vi "LAS-CTS_TargetScanner.vi"() -> ()   [LabVIEW 2024]
doc: "Shows how to move a motor to an absolute position."
uses:
  E:/E-book/LAS/LAS DAQ/LAS LV Scan/Kinesis/Thorlabs.MotionControl.Controls.dll
  Kinesis/Thorlabs.MotionControl.Controls.dll
  <vilib>/Analysis/baseanly.llb/Mean (DBL).vi
  E:/E-book/LAS/LAS DAQ/LAS LV Scan/Kinesis/ThorLabs.MotionControl.KCube.DCServoCLI.dll
  Kinesis/ThorLabs.MotionControl.KCube.DCServoCLI.dll
  <vilib>/httpClient/LabVIEWHTTPClient.lvlib
  <vilib>/Analysis/NI_AALBase.lvlib
panel:
  out "Filename":path
  in  "File #":i32 format="%03d"
  in  "base filename":string
  in  "Filepath":path
  in  "Target ID":string
  out "Last Spot Charge (pC)":dbl
  out "Laser Energy (uJ)":dbl format="%#.3f"
  out "Pulses Remaining":i32
  out "Laser On/Off":bool
  in  "Energy Meter VISA port":refnum<visa-resource-name>="IntegraEnergyMeter"
  in  "Keithley VISA port":refnum<visa-resource-name>="Keithly6514"
  out "Scan Graph":dbl[][](graph)
  in  "KCubeDCServoControl Z axis":refnum<k24>(container)
  in  "KCubeDCServoControl X axis":refnum<k24>(container)
  out "K6514 Error":errorcluster
  out "Time Remaining (min)":dbl format="%#_2f"
  out "sec per spot":dbl
  out "scan started":bool
  out "Scan Progress":u8(slide) scale=0.0..42.0
  out "Scan Time (hr)":dbl format="%#_2f"
  in  "Number of Laser Pulses":i32=100
  in  "X Start Position":dbl=5.0
  in  "Z Start Position":dbl=4.0
  in  "Z Step Size (um)":dbl=500.0
  in  "# of Z Positions":i32=2
  in  "# of X Positions":i32=2
  in  "X Step Size (um)":dbl=500.0
  in  "Start Scan":bool
  out "CurrentPosZ":dbl=6.0
  out "CurrentPosX":dbl=6.0
  in  "SerialNumber Z":string="27261646"
  in  "SerialNumber X":string="27261828"
  # "Connection Setup"
  # "Scan Parameters"
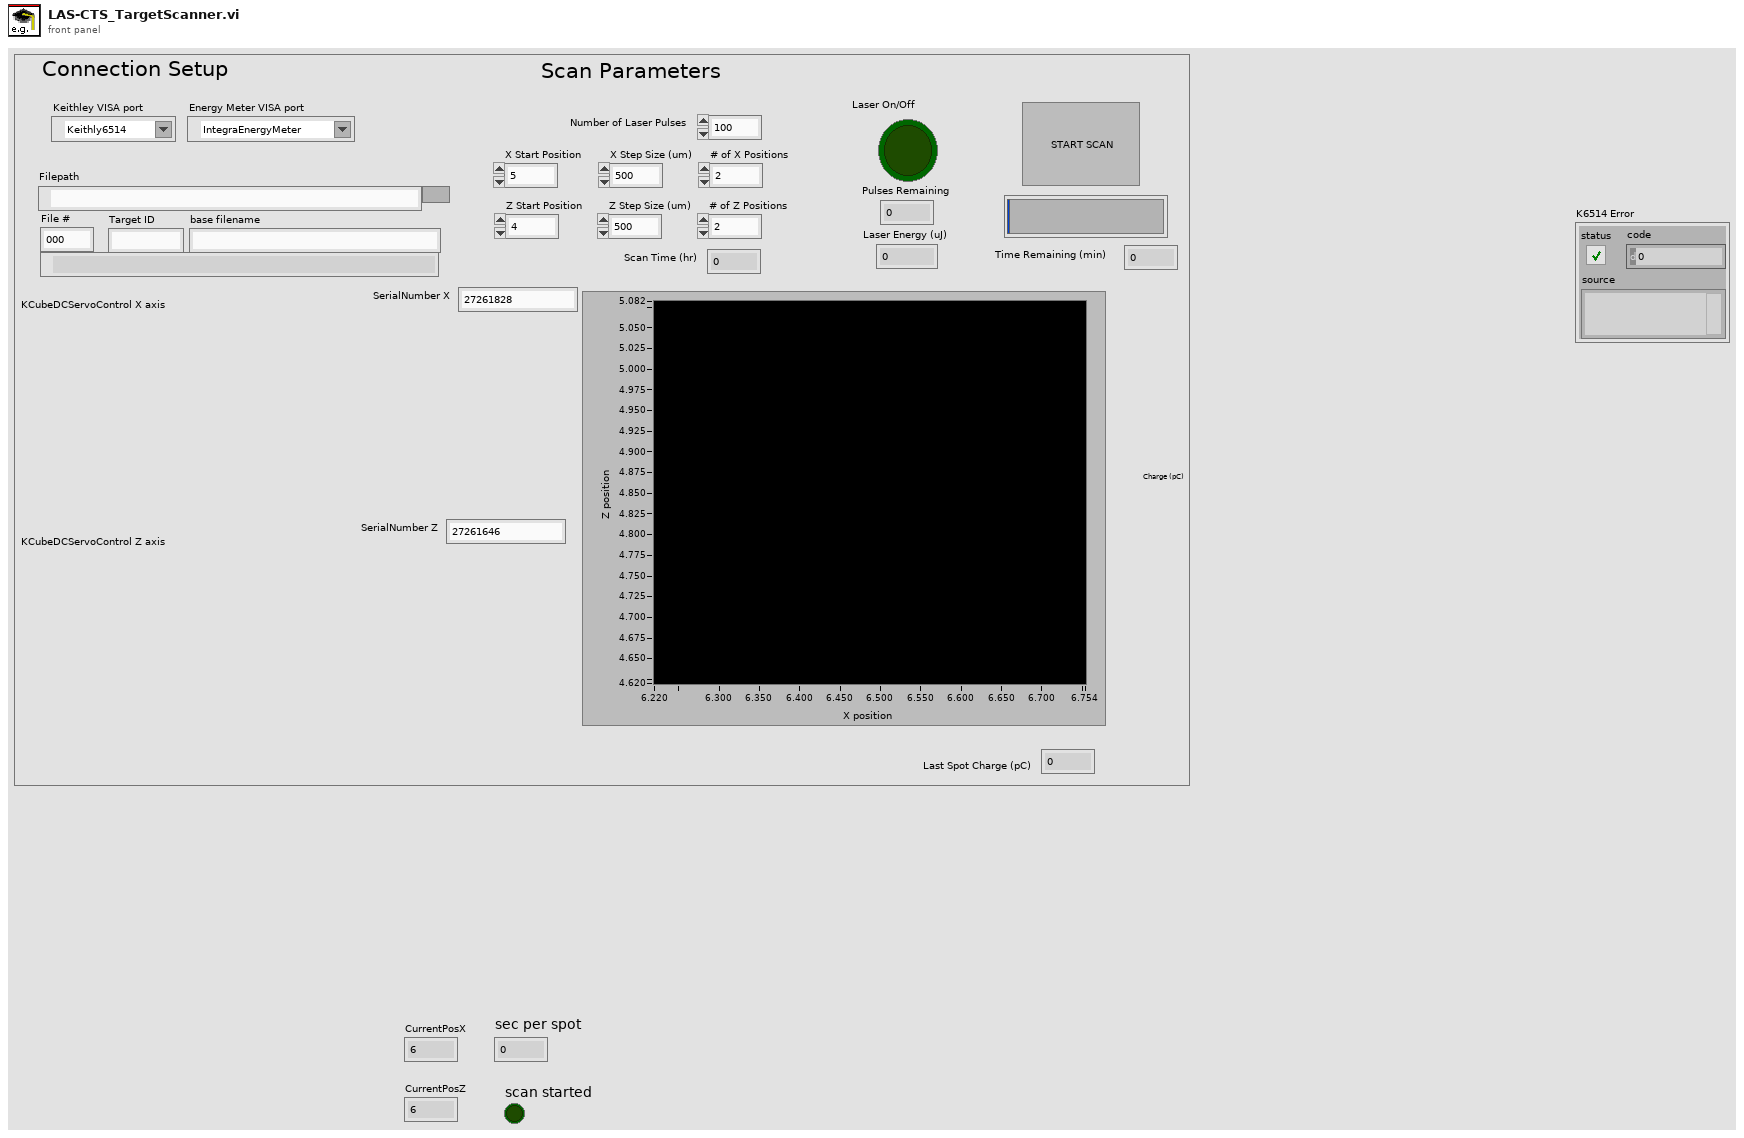
[diagram p1: front panel]
types:
  T1 = enum16{"open", "replace", "create", "open or create", "replace or create", "replace or create with confirmation"}
  T2 = typedef "LabVIEWHTTPClient.lvlib/ClientHandle.ctl" = refnum<k1>
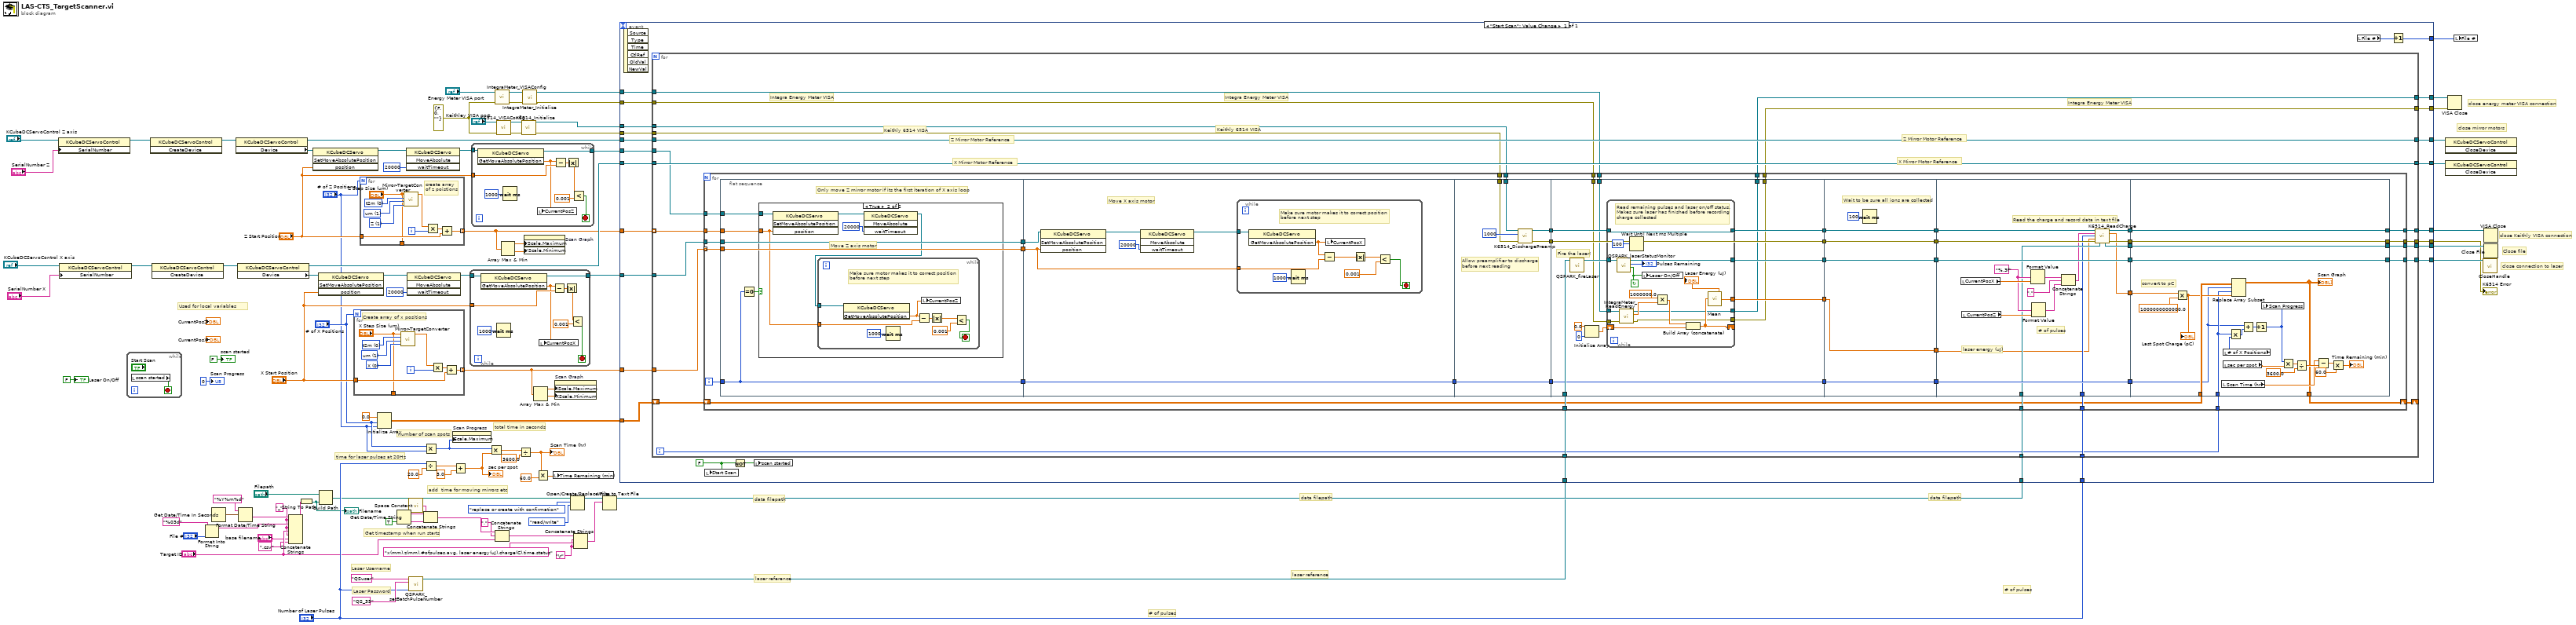
[diagram p0: block diagram]
diagram:
  w7 = "_" ("string")
  w32 = errorcluster {"status"=FALSE, "code"=0, "source"=""} ("error in (no error)")
  w25 = "\r"
  # "Get timestamp when run starts"
  # "close energy meter VISA connection"
  # "total time in seconds"
  # "add  time for moving mirrors etc"
  # "number of scan spots"
  # "time for laser pulses at 20Hz"
  # "data filepath"
  # "data filepath"
  # "close Keithly VISA connection"
  # "close mirror motors"
  # "close connection to laser"
  # "Close file"
  # "Used for local variables"
  # "data filepath"
  # "laser reference"
  # "# of pulses"
  # "# of pulses"
  # "laser reference"
  # "Laser Password"
  # "Laser Username"
  n1 = property class="KCubeDCServoControl"(reference="KCubeDCServoControl Z axis", "SerialNumber"="SerialNumber Z") -> (reference out=w94:refnum<k24>)  [unwired: 1 in, 1 out]
  n2 = property class="KCubeDCServoControl"(reference="KCubeDCServoControl X axis", "SerialNumber"="SerialNumber X") -> (reference out=w97:refnum<k24>)  [unwired: 1 in, 1 out]
  n3 = while {
    stop <- w98 stop-if-true
    n4 = local read "scan started"() -> (w98:bool)
  }
  n5 = invoke class="KCubeDCServoControl" method="CreateDevice"(reference=w94) -> (reference out=w88:refnum<k24>)  [unwired: 2 in, 2 out]
  n6 = invoke class="KCubeDCServoControl" method="CreateDevice"(reference=w97) -> (reference out=w95:refnum<k24>)  [unwired: 2 in, 2 out]
  n7 = Format Into String(format string="%03d", "File #") -> (resulting string=w10:string)  [unwired: 2 in, 1 out]
  n8 = Get Date/Time In Seconds() -> (seconds since 1Jan1904=w15:timestamp)
  n9 = property class="KCubeDCServoControl"(reference=w88) -> (reference out=w85:refnum<k24>, "Device"=w1:refnum<k24>)  [unwired: 1 in, 1 out]
  n10 = property class="KCubeDCServoControl"(reference=w95) -> (reference out=w84:refnum<k24>, "Device"=w76:refnum<k24>)  [unwired: 1 in, 1 out]
  n11 = Format Date/Time String(time format string (%c)="%Y%m%d", seconds (now)=w15) -> (date/time string=w13:string)  [unwired: 1 in]
  n12 = Concatenate Strings(w13, w7, w10, w7, "Target ID", w7, "base filename", ".csv" ("string")) -> (w16:string)
  n13 = String To Path(string=w16) -> (path=w3:path)
  "Filename" <- w3
  n14 = invoke class="KCubeDCServo" method="SetMoveAbsolutePosition"(reference=w1, "position"="Z Start Position") -> (reference out=w80:refnum<k24>)  [unwired: 2 in, 3 out]
  n15 = invoke class="KCubeDCServo" method="SetMoveAbsolutePosition"(reference=w76, "position"="X Start Position") -> (reference out=w78:refnum<k24>)  [unwired: 2 in, 3 out]
  n16 = Build Path(base path="Filepath", name or relative path=w3) -> (appended path=w9:path)
  n17 = for {
    N: "# of X Positions" -> [_]
    tunnel: [w103] -> w53 mode=indexing
    tunnel: "X Start Position" -> [w100]
    tunnel: ["X Step Size (um)"] -> _
    i -> [w101]
    w107 = u16 0 items=["X", "Z"] ("axis")
    w105 = u16 0 items=["t2m", "m2t"] ("Conversion")
    w106 = u16 1 items=["mm", "um"] ("input units")
    # "Create array of x positions"
    n18 = call "Mirror-TargetConverter.vi"("axis"=w107, "input units"=w106, "Conversion"=w105, "input distance"="X Step Size (um)") -> ("output distance"=w102:dbl)  [unwired: 7 in]
    n19 = Multiply(x=w102, y=w101) -> (x*y=w104:dbl)
    n20 = Add(x=w104, y=w100) -> (x+y=w103:dbl)
  }
  n21 = for {
    N: "# of Z Positions" -> [_]
    tunnel: [w110] -> w54 mode=indexing
    tunnel: "Z Start Position" -> [w109]
    tunnel: ["Z Step Size (um)"] -> _
    i -> [w116]
    w114 = u16 1 items=["X", "Z"] ("axis")
    w113 = u16 0 items=["t2m", "m2t"] ("Conversion")
    w115 = u16 1 items=["mm", "um"] ("input units")
    # "create array\nof z poistions"
    n22 = call "Mirror-TargetConverter.vi"("axis"=w114, "input units"=w115, "Conversion"=w113, "input distance"="Z Step Size (um)") -> ("output distance"=w112:dbl)  [unwired: 7 in]
    n23 = Multiply(x=w112, y=w116) -> (x*y=w111:dbl)
    n24 = Add(x=w111, y=w109) -> (x+y=w110:dbl)
  }
  n25 = Initialize Array(0.0, "# of X Positions", "# of Z Positions") -> (w34:dbl[][])
  n26 = Get Date/Time String(want seconds? (F)=TRUE) -> (date string=w24:string, time string=w23:string)  [unwired: 2 in]
  n27 = invoke class="KCubeDCServo" method="MoveAbsolute"(reference=w80, "waitTimeout"=20000) -> (reference out=w72:refnum<k24>)  [unwired: 2 in, 3 out]
  n28 = invoke class="KCubeDCServo" method="MoveAbsolute"(reference=w78, "waitTimeout"=20000) -> (reference out=w75:refnum<k24>)  [unwired: 2 in, 3 out]
  n29 = call <vilib>:"Space Constant.vi"() -> ("String"=w22:string)
  n30 = call "QSPARK_setBatchPulseNumber.vi"("Number of Pulses"="Number of Laser Pulses", "password"="QS_35", "username"="QSuser") -> ("client handle out"=w68:T2)  [unwired: 8 in]
  n31 = Multiply(x="# of X Positions", y="# of Z Positions") -> (x*y=w52:i32)
  n32 = Divide(x="Number of Laser Pulses", y=20.0) -> (x/y=w59:dbl)
  n33 = Concatenate Strings(w24, w22, w23) -> (w20:string)
  n34 = property on="Scan Progress" class="Slide (strict)"("Scale.Maximum"=w52) -> ()  [unwired: 2 in, 2 out]
  n35 = Add(x=w59, y=3.0) -> (x+y=w57:dbl)
  "sec per spot" <- w57
  n36 = while {
    tunnel: w75 -> [w125]
    tunnel: "X Start Position" -> [w123]
    tunnel: [w122] -> w73
    stop <- w119 stop-if-true
    n37 = invoke class="KCubeDCServo" method="GetMoveAbsolutePosition"(reference=w125) -> (reference out=w122:refnum<k24>, "GetMoveAbsolutePosition"=w117:dbl)  [unwired: 2 in, 1 out]
    n38 = Wait (ms)(milliseconds to wait=u32 1000) -> ()  [unwired: 1 out]
    n39 = local write "CurrentPosX"(w117) -> ()
    n40 = Subtract(x=w117, y=w123) -> (x-y=w118:dbl)
    n41 = Absolute Value(x=w118) -> (abs(x)=w121:dbl)
    n42 = Less?(x=w121, y=0.001) -> (x < y?=w119:bool)
  }
  n43 = while {
    tunnel: w72 -> [w134]
    tunnel: "Z Start Position" -> [w130]
    tunnel: [w127] -> w71
    stop <- w132 stop-if-true
    n44 = invoke class="KCubeDCServo" method="GetMoveAbsolutePosition"(reference=w134) -> (reference out=w127:refnum<k24>, "GetMoveAbsolutePosition"=w129:dbl)  [unwired: 2 in, 1 out]
    n45 = Wait (ms)(milliseconds to wait=u32 1000) -> ()  [unwired: 1 out]
    n46 = local write "CurrentPosZ"(w129) -> ()
    n47 = Subtract(x=w129, y=w130) -> (x-y=w126:dbl)
    n48 = Absolute Value(x=w126) -> (abs(x)=w133:dbl)
    n49 = Less?(x=w133, y=0.001) -> (x < y?=w132:bool)
  }
  n50 = Multiply(x=w52, y=w57) -> (x*y=w56:dbl)
  n51 = call "IntegraMeter_VISAConfig.vi"("error in (no error)"=w32, "VISA resource name"="Energy Meter VISA port") -> ("error out"=w31:errorcluster, "reference out"=w30:refnum<visa-resource-name>)  [unwired: 8 in]
  n52 = Concatenate Strings(w20, "," ("string"), "Target ID") -> (w18:string)
  n53 = call "K6514_VISAConfig.vi"("error in (no error)"=w32, "VISA resource name"="Keithley VISA port") -> ("error out"=w41:errorcluster, "reference out"=w40:refnum<visa-resource-name>)  [unwired: 8 in]
  n54 = Array Max & Min(array=w54) -> (max value=w47:dbl, min value=w46:dbl)  [unwired: 2 out]
  n55 = Divide(x=w56, y=3600.0) -> (x/y=w44:dbl)
  "Scan Time (hr)" <- w44
  n56 = call "K6514_Initialize.vi"("error in (no error)"=w41, "VISA resource name"=w40) -> ("error out"=w38:errorcluster, "VISA resource name out"=w39:refnum<visa-resource-name>)  [unwired: 8 in]
  n57 = call "IntegraMeter_Initialize.vi"("error in"=w31, "VISA resource name"=w30) -> ("error out"=w28:errorcluster, "VISA resource name out"=w29:refnum<visa-resource-name>)  [unwired: 8 in]
  n58 = property on="Scan Graph" class="IntGraph (strict)"("YScale.Maximum"=w47, "YScale.Minimum"=w46) -> ()  [unwired: 2 in, 2 out]
  n59 = Array Max & Min(array=w53) -> (max value=w49:dbl, min value=w48:dbl)  [unwired: 2 out]
  n60 = Multiply(x=w44, y=60.0) -> (x*y=w45:dbl)
  n61 = local write "Time Remaining (min)"(w45) -> ()
  n62 = property on="Scan Graph" class="IntGraph (strict)"("XScale.Maximum"=w49, "XScale.Minimum"=w48) -> ()  [unwired: 2 in, 2 out]
  n63 = Open/Create/Replace File(file path (use dialog)=w9, operation (0:open)=T1."replace or create with confirmation", access (0:read/write)=enum16{"read/write", "read-only", "write-only"}."read/write") -> (refnum out=w90:refnum<file>)  [unwired: 3 in, 2 out]
  n64 = Concatenate Strings(w18, w25, "x(mm),z(mm),#ofpulses,avg. laser energy(uJ),charge(C),time,status", w25) -> (w81:string)
  n65 = Write to Text File(file (use dialog)=w90, text=w81) -> (refnum out=w89:refnum<file>)  [unwired: 2 in, 2 out]
  n66 = event shown="[0] \"Start Scan\": Value Change" {
    selector: _ -> [_]
    dyn-events: _ -> [_]
    timeout: _ -> [_]
    tunnel: [w160] -> w93
    tunnel: w89 -> [w159]
    tunnel: w53 -> [w158]
    tunnel: [w157] -> w87
    tunnel: [w156] -> w86
    tunnel: w85 -> [w155]
    tunnel: w84 -> [w154]
    tunnel: [w153] -> w83
    tunnel: w73 -> [w152]
    tunnel: w71 -> [w151]
    tunnel: w39 -> [w150]
    tunnel: w68 -> [w149]
    tunnel: "Number of Laser Pulses" -> [w148]
    tunnel: [w147] -> w67
    tunnel: w34 -> [w146]
    tunnel: w54 -> [w145]
    tunnel: w38 -> [w142]
    tunnel: [w141] -> w37
    tunnel: w29 -> [w140]
    tunnel: w28 -> [w139]
    tunnel: [w138] -> w27
    tunnel: [w137] -> w26
    tunnel: [w135] -> w4
    event "Start Scan": Value Change {
      w143 = FALSE
      n67 = event-data() -> ()  [unwired: 1 in, 6 out]
      n68 = for {
        tunnel: w152 -> [w182]
        tunnel: w145 -> [w173] mode=indexing
        tunnel: [w181] -> w160
        tunnel: w159 -> [w180]
        tunnel: w148 -> [w179]
        tunnel: w158 -> [w178]
        tunnel: [w177] -> w157
        tunnel: [w176] -> w156
        tunnel: w155 -> [w177]
        tunnel: w154 -> [w176]
        tunnel: [w175] -> w153
        tunnel: w151 -> [w172]
        tunnel: w149 -> [w174]
        tunnel: w150 -> [w171]
        tunnel: [w170] -> w147
        shift-right: [w167] -> _
        shift-left: w146 -> [w168]
        tunnel: w142 -> [w166]
        tunnel: [w165] -> w141
        tunnel: w140 -> [w164]
        tunnel: w139 -> [w163]
        tunnel: [w162] -> w138
        tunnel: [w161] -> w137
        i -> [w169]
        # "Integra Energy Meter VISA"
        # "Integra Energy Meter VISA"
        # "Integra Energy Meter VISA"
        # "Keithly 6514 VISA"
        # "X Mirror Motor Reference"
        # "X Mirror Motor Reference"
        # "Z Mirror Motor Reference"
        # "Keithly 6514 VISA"
        # "Z Mirror Motor Reference"
        n69 = for {
          tunnel: w182 -> [w226]
          tunnel: w178 -> [w225] mode=indexing
          tunnel: [w224] -> w181
          tunnel: w180 -> [w222]
          tunnel: w179 -> [w221]
          tunnel: [w209] -> w175
          tunnel: w174 -> [w220]
          tunnel: w173 -> [w213]
          tunnel: w172 -> [w212]
          tunnel: w171 -> [w210]
          tunnel: [w208] -> w170
          tunnel: w169 -> [w200]
          shift-right: [w198] -> w167
          shift-left: w168 -> [w199]
          tunnel: w166 -> [w197]
          tunnel: [w191] -> w165
          tunnel: w164 -> [w187]
          tunnel: w163 -> [w186]
          tunnel: [w185] -> w162
          tunnel: [w184] -> w161
          i -> [w211]
          n70 = flat-sequence {
            tunnel: w225 -> [w228]
            tunnel: w226 -> [w229]
            tunnel: [w229] -> w215
            tunnel: [w228] -> w214
            tunnel: w213 -> [w232]
            tunnel: w212 -> [w231]
            tunnel: w211 -> [w227]
            tunnel: [w227] -> w201
            tunnel: w214 -> [w250]
            tunnel: w215 -> [w249]
            tunnel: [w246] -> w202
            tunnel: w201 -> [w246]
            tunnel: [w264] -> w223
            tunnel: w210 -> [w263]
            tunnel: [w265] -> w203
            tunnel: w202 -> [w265]
            tunnel: w197 -> [w261]
            tunnel: [w260] -> w195
            tunnel: [w280] -> w219
            tunnel: [w279] -> w217
            tunnel: w223 -> [w278]
            tunnel: w220 -> [w277]
            tunnel: [w275] -> w204
            tunnel: w203 -> [w275]
            tunnel: w195 -> [w274]
            tunnel: [w274] -> w194
            tunnel: [w270] -> w189
            tunnel: w187 -> [w269]
            tunnel: w186 -> [w268]
            tunnel: [w267] -> w185
            tunnel: [w266] -> w184
            tunnel: w219 -> [w302]
            tunnel: [w302] -> w218
            tunnel: w217 -> [w301]
            tunnel: [w301] -> w216
            tunnel: [w299] -> w205
            tunnel: w204 -> [w299]
            tunnel: w194 -> [w298]
            tunnel: [w298] -> w193
            tunnel: w189 -> [w297]
            tunnel: [w297] -> w188
            tunnel: w218 -> [w311]
            tunnel: w216 -> [w320]
            tunnel: w222 -> [w307]
            tunnel: w221 -> [w305]
            tunnel: [w320] -> w207
            tunnel: [w313] -> w206
            tunnel: w205 -> [w313]
            tunnel: [w312] -> w196
            tunnel: w193 -> [w310]
            tunnel: [w303] -> w192
            tunnel: [w309] -> w190
            tunnel: w188 -> [w304]
            tunnel: [w308] -> w183
            tunnel: [w341] -> w208
            tunnel: [w342] -> w209
            tunnel: [w343] -> w224
            tunnel: w207 -> [w343]
            tunnel: w206 -> [w334]
            tunnel: w200 -> [w336]
            tunnel: w199 -> [w340]
            tunnel: [w326] -> w198
            tunnel: w196 -> [w341]
            tunnel: w192 -> [w339]
            tunnel: [w321] -> w191
            tunnel: w190 -> [w321]
            tunnel: w183 -> [w342]
            frame #0 {
              # "Only move Z mirror motor if its the first iteration of X axis loop"
              n71 = Equal To 0?(x=w227) -> (x = 0?=w230:bool)
              n72 = case shown="True" w230 {
                tunnel: w232 -> [_ w235]
                tunnel: w231 -> [_ w234]
                frame False {
                }
                frame True {
                  # "Move Z axis motor"
                  n73 = invoke class="KCubeDCServo" method="SetMoveAbsolutePosition"(reference=w234, "position"=w235) -> (reference out=w237:refnum<k24>)  [unwired: 2 in, 3 out]
                  n74 = invoke class="KCubeDCServo" method="MoveAbsolute"(reference=w237, "waitTimeout"=20000) -> (reference out=w233:refnum<k24>)  [unwired: 2 in, 3 out]
                  n75 = while {
                    tunnel: w235 -> [w242]
                    tunnel: w233 -> [w238]
                    stop <- w243 stop-if-true
                    # "Make sure motor makes it to correct position\nbefore next step"
                    n76 = invoke class="KCubeDCServo" method="GetMoveAbsolutePosition"(reference=w238) -> ("GetMoveAbsolutePosition"=w239:dbl)  [unwired: 2 in, 2 out]
                    n77 = Wait (ms)(milliseconds to wait=u32 1000) -> ()  [unwired: 1 out]
                    n78 = Subtract(x=w239, y=w242) -> (x-y=w240:dbl)
                    n79 = local write "CurrentPosZ"(w239) -> ()
                    n80 = Absolute Value(x=w240) -> (abs(x)=w244:dbl)
                    n81 = Less?(x=w244, y=0.001) -> (x < y?=w243:bool)
                  }
                }
              }
            }
            frame #1 {
              # "Move X axis motor"
              n82 = invoke class="KCubeDCServo" method="SetMoveAbsolutePosition"(reference=w249, "position"=w250) -> (reference out=w248:refnum<k24>)  [unwired: 2 in, 3 out]
              n83 = invoke class="KCubeDCServo" method="MoveAbsolute"(reference=w248, "waitTimeout"=20000) -> (reference out=w251:refnum<k24>)  [unwired: 2 in, 3 out]
              n84 = while {
                tunnel: w251 -> [w258]
                tunnel: w250 -> [w256]
                stop <- w254 stop-if-true
                # "Make sure motor makes it to correct position\nbefore next step"
                n85 = invoke class="KCubeDCServo" method="GetMoveAbsolutePosition"(reference=w258) -> ("GetMoveAbsolutePosition"=w252:dbl)  [unwired: 2 in, 2 out]
                n86 = Wait (ms)(milliseconds to wait=u32 1000) -> ()  [unwired: 1 out]
                n87 = Subtract(x=w252, y=w256) -> (x-y=w257:dbl)
                n88 = local write "CurrentPosX"(w252) -> ()
                n89 = Absolute Value(x=w257) -> (abs(x)=w255:dbl)
                n90 = Less?(x=w255, y=0.001) -> (x < y?=w254:bool)
              }
            }
            frame #2 {
              # "Allow preamplifier to discharge\nbefore next reading"
              n91 = call "K6514_DischargePreamp.vi"("error in (no error)"=w261, "discharge time (ms)"=u32 1000 ("milliseconds to wait"), "VISA resource name in"=w263) -> ("error out"=w260:errorcluster, "VISA resource name out"=w264:refnum<visa-resource-name>)  [unwired: 7 in]
            }
            frame #3 {
              # "Fire the laser!"
              n92 = call "QSPARK_fireLaser.vi"("client handle"=w277) -> ("client handle out"=w276:T2)  [unwired: 10 in]
              n93 = Initialize Array(0.0 ("element"), 0 ("dimension size")) -> (w271:dbl[])
              n94 = while {
                tunnel: w278 -> [w295]
                tunnel: [w295] -> w280
                tunnel: w276 -> [w294]
                tunnel: [w293] -> w279
                shift-right: [w287] -> _
                shift-left: w271 -> [w290]
                tunnel: [w285] -> w270
                tunnel: w269 -> [w284]
                tunnel: w268 -> [w283]
                tunnel: [w282] -> w267
                tunnel: [w281] -> w266
                stop <- w291 continue-if-true
                # "Read remaining pulses and laser on/off status. \nMakes sure laser has finished before recording \ncharge collected"
                n95 = call "QSPARK_laserStatusMonitor.vi"("client handle"=w294) -> ("laser on?"=w291:bool, "remaining pulses"=→"Pulses Remaining":i32, "client handle out"=w293:T2)  [unwired: 8 in]
                n96 = call "IntegraMeter_ReadEnergy.vi"("error in (no error)"=w283, "VISA resource name"=w284) -> ("error out"=w281:errorcluster, "Laser Energy (J)"=w288:dbl, "VISA resource name out"=w282:refnum<visa-resource-name>)  [unwired: 7 in]
                n97 = Wait Until Next ms Multiple(millisecond multiple=u32 100) -> ()  [unwired: 1 out]
                n98 = local write "Laser On/Off"(w291) -> ()
                n99 = Multiply(x=1000000.0, y=w288) -> (x*y=w286:dbl)
                n100 = Build Array (concatenate)(w286, w290) -> (w287:dbl[])
                n101 = call-poly <vilib>:"Mean.vi"("X"=w287) -> ("mean"=w285:dbl)  [unwired: 1 out]
                "Laser Energy (uJ)" <- w285
              }
            }
            frame #4 {
              # "Wait to be sure all ions are collected"
              n102 = Wait (ms)(milliseconds to wait=u32 100) -> ()  [unwired: 1 out]
            }
            frame #5 {
              w314 = "%.3f" ("format string")
              # "laser energy (uJ)"
              # "Read the charge and record data in text file"
              # "# of pulses"
              n103 = local read "CurrentPosX"() -> (w316:dbl)
              n104 = local read "CurrentPosZ"() -> (w315:dbl)
              n105 = Format Value(format string=w314, value (0)=w316) -> (output string=w319:string)  [unwired: 1 in]
              n106 = Format Value(format string=w314, value (0)=w315) -> (output string=w318:string)  [unwired: 1 in]
              n107 = Concatenate Strings(w319, ",", w318) -> (w306:string)
              n108 = call "K6514_ReadCharge.vi"("VISA resource name"=w311, "position"=w306, "Number of Pulses"=w305, "Laser Energy (uJ)"=w304, "error in (no error)"=w310, "file refnum"=w307) -> ("VISA resource name out"=w312:refnum<visa-resource-name>, "charge(C)"=w303:dbl, "file refnum out"=w308:refnum<file>, "error out"=w309:errorcluster)  [unwired: 5 in, 1 out]
            }
            frame #6 {
              # "convert to pC"
              n109 = Multiply(x=w339, y=1000000000000.0) -> (x*y=w337:dbl)
              "Last Spot Charge (pC)" <- w337
              n110 = local read "Scan Time (hr)"() -> (w327:dbl)
              n111 = local read "# of X Positions"() -> (w332:i32)
              n112 = local read "sec per spot"() -> (w331:dbl)
              n113 = Multiply(x=w336, y=w332) -> (x*y=w335:i32)
              n114 = Replace Array Subset(array=w340, new element=w337, index (row)=w334, index (col)=w336) -> (w326:dbl[][])
              "Scan Graph" <- w326
              n115 = Add(x=w334, y=w335) -> (x+y=w333:i32)
              n116 = Increment(x=w333) -> (x+1=w325:i32)
              n117 = local write "Scan Progress"(w325) -> ()
              n118 = Multiply(x=w325, y=w331) -> (x*y=w330:dbl)
              n119 = Divide(x=w330, y=3600.0) -> (x/y=w328:dbl)
              n120 = Subtract(x=w327, y=w328) -> (x-y=w324:dbl)
              n121 = Multiply(x=w324, y=60.0) -> (x*y=→"Time Remaining (min)":dbl)
            }
          }
        }
      }
      n122 = local write "Start Scan"(w143) -> ()
      n123 = Not(x=w143) -> (.not. x?=w144:bool)
      n124 = local write "scan started"(w144) -> ()
      n125 = local read "File #"() -> (w136:i32)
      n126 = Increment(x=w136) -> (x+1=w135:i32)
    }
  }
  "K6514 Error" <- w37
  n127 = invoke class="KCubeDCServoControl" method="CloseDevice"(reference=w87) -> ()  [unwired: 2 in, 3 out]
  n128 = invoke class="KCubeDCServoControl" method="CloseDevice"(reference=w86) -> ()  [unwired: 2 in, 3 out]
  n129 = VISA Close(VISA resource name=w27, error in (no error)=w26) -> ()  [unwired: 1 out]
  n130 = local write "File #"(w4) -> ()
  n131 = call <vilib>:"CloseHandle.vi"("client handle"=w93) -> ()  [unwired: 14 in, 1 out]
  n132 = VISA Close(VISA resource name=w67) -> ()  [unwired: 1 in, 1 out]
  n133 = Close File(refnum=w83) -> ()  [unwired: 1 in, 2 out]
  "Laser On/Off" <- FALSE ("Laser On/Off")
  "scan started" <- FALSE
  "Scan Progress" <- u8 0 ("Scan Progress")
